vi "CircleMath.vi"(1 "Target Heading":dbl, 2 "Current Heading":dbl) -> (0 "Delta Heading":dbl)   [LabVIEW 2014]
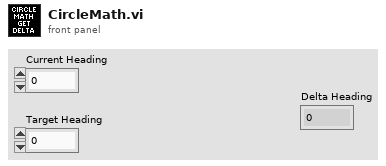
[diagram p1: front panel]
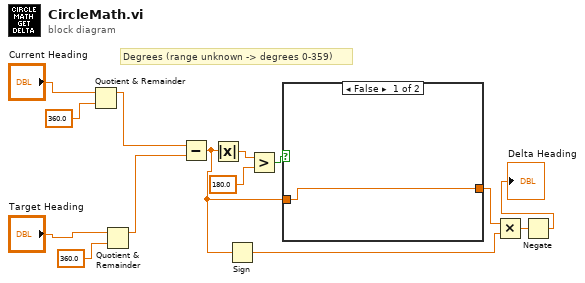
[diagram p0: block diagram]
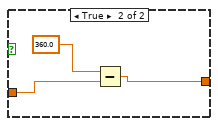
[diagram p2: hidden frame]
diagram:
  # "Degrees (range unknown -> degrees 0-359)"
  n1 = Quotient & Remainder(x="Current Heading", y=360.0) -> (x-y*floor(x/y)=w10:dbl)  [unwired: 1 out]
  n2 = Quotient & Remainder(x="Target Heading", y=360.0) -> (x-y*floor(x/y)=w9:dbl)  [unwired: 1 out]
  n3 = Subtract(x=w10, y=w9) -> (x-y=w5:dbl)
  n4 = Absolute Value(x=w5) -> (abs(x)=w8:dbl)
  n5 = Sign(1:w5) -> (0:w3:dbl)
  n6 = Greater?(x=w8, y=180.0) -> (0:w6:bool)
  n7 = case shown="False" w6 {
    tunnel: w5 -> [w15 w17]
    tunnel: [w15 w16] -> w4
    frame False {
    }
    frame True {
      n8 = Subtract(x=360.0, y=w17) -> (x-y=w16:dbl)
    }
  }
  n9 = Multiply(x=w4, y=w3) -> (x*y=w2:dbl)
  n10 = Negate(x=w2) -> (-x=→"Delta Heading":dbl)
